vi "Expt5_MT FSK Transceiver_Student_lab.vi"(0 "# Message Symbols":i32=1000, 5 "Eb/N0, dB":dbl(slide)=80.0 scale=0.0..100.0, 9 "Symbol Phase Continuity":enum16{"continuous", "discontinuous"}(ring), 11 "Reset ? (T)":bool=TRUE, 14 "?":T3(tab)=enum."Eye diagram (RX)") -> (3 "FSK System Parameters":T2={"samples per symbol (16)"=4, "symbol map"=[-25000.0, 25000.0], "symbol phase continuity"=enum."continuous"} {"symbol map" format="%.2f"}, 4 "Output Complex Waveform":cluster{"t0":dbl, "dt":dbl, "Y":cdb[]} {"Y" format="%.3f"; "dt" format="%^.2e"; "t0" format="%.4f"}, 6 "Transmitted  Bits":i8[](array[numeric]), 8 "Received Bits":i8[](array[numeric]), 10 "Bit Error Rate":dbl format="%.4e", 13 "Last Sync Found Index":dbl format="%.4f", 15 "Error Out":errorcluster)   [LabVIEW 2020]
doc: "This example demonstrates generation and analysis of FSK modulated signals. You can specify transmit filter parameters, Eb/No, and frequency offset. This example demonstrates programming techniques for resetting the transmitter in cases where the receiver (demodulator) lock is lost. You can also view results of the demodulation on an eye diagram and perform measurements such as bit error rate."
uses:
  <vilib>/addons/Modulation/niDMT.lvlib
  <vilib>/addons/Modulation/niAMT.lvlib
  <vilib>/addons/Modulation/Digital/Support/Controls/FSK System Parameters.ctl
panel:
  out "Estimated Eb/N0(dB)":dbl
  in  "BT":dbl=0.5 format="%.2f"
  out "Current Sampling Rate":dbl=400000.0 format="%.2p"
  in  "Symbol Rate":dbl=100000.0 format="%.2p"
  out "Frequency Offset (Hz)":dbl=-5.3151869530752014e-05 format="%.2f"
  in  "Frequency Offset (Hz)":dbl(slide) scale=-1000.0..1000.0
  in  "FSK Deviation (Hz)":dbl=25000.0 format="%.2p"
  in  "M-FSK":enum16{"2", "4", "8", "16", "32", "64"}(ring)
  in  "TX Filter":T1(ring)=enum."Gaussian"
  out "BER Trigger Found":bool
  in  "Stop":bool
  out "TX Symbols":T4(graph)={{"1/x"=0.0, 1e-05, [1, 1, 0, 1, 0, 1, 1, 0, 1, 0, 0, 1, 1, 1, 1, 1, 1, 1, 0, 1, 0, 0, 0, 1, 0, 1, 1, 0, 0, 0, 1, 1, 1, 0, 1, 0, 1, 1, 0, 0, 1, 0, 1, 1, 0, 0, 1, 1, 1, 1, 0, 0, 0, 1, 1, 1, 1, 1, 0, 1, 1, 1, 0, 1, 0, 0, 0, 0, 0, 1, 1, 0, 1, 0, 1, 1, 0, 1, 1, 0, 1, 1, 1, 0, 1, 1, 0, 0, 0, 0, 0, 1, 0, 1, 1, 0, 1, 0, 1, 1, 1, 1, 1, 0, 1, 0, 1, 0, 1, 0, 1, 0, 0, 0, 0, 0, 0, 1, 0, 1, 0, 0, 1, 0, 1, 0, 1, 1, 1, 1, 0, 0, 1, 0, 1, 1, 1, 0, 1, 1, 1, 0, 0, 0, 0, 0, 0, 1, 1, 1, 0, 0, 1, 1, 1, 0, 1, 0, 0, 1, 0, 0, 1, 1, 1, 1, 0, 1, 0, 1, 1, 1, 0, 1, 0, 1, 0, 0, 0, 1, 0, 0, 1, 0, 0, 0, 0, 1, 1, 0, 0, 1, 1, 1, 0, 0, 0, 0, 1, 0, 1, 1, 1, 1, 0, 1, 1, 0, 1, 1, 0, 0, 1, 1, 0, 1, 0, 0, 0, 0, 1, 1, 1, 0, 1, 1, 1, 1, 0, 0, 0, 0, 1, 1, 1, 1, 1, 1, 1, 1, 1, 0, 0, 0, 0, 0, 1, 1, 1, 1, 0, 1, 1, 1, 1, 1, 0, 0, 0, 1, 0, 1, 1, 1, 0, 0, 1, 1, 0, 0, 1, 0, 0, 0, 0, 0, 1, 0, 0, 1, 0, 1, 0, 0, 1, 1, 1, 0, 1, 1, 0, 1, 0, 0, 0, 1, 1, 1, 1, 0, 0, 1, 1, 1, 1, 1, 0, 0, 1, 1, 0, 1, 1, 0, 0, 0, 1, 0, 1, 0, 1, 0, 0, 1, 0, 0, 0, 1, 1, 1, 0, 0, 0, 1, 1, 0, 1, 1, 0, 1, 0, 1, 0, 1, 1, 1, 0, 0, 0, 1, 0, 0, 1, 1, 0, 0, 0, 1, 0, 0, 0, 1, 0, 0, 0, 0, 0, 0, 0, 0, 1, 0, 0, 0, 0, 1, 0, 0, 0, 1, 1, 0, 0, 0, 0, 1, 0, 0, 1, 1, 1, 0, 0, 1, 0, 1, 0, 1, 0, 1, 1, 0, 0, 0, 0, 1, 1, 0, 1, 1, 1, 1, 0, 1, 0, 0, 1, 1, 0, 1, 1, 1, 0, 0, 1, 0, 0, 0, 1, 0, 1, 0, 0, 0, 0, 1, 0, 1, 0, 1, 1, 0, 1, 0, 0, 1, 1, 1, 1, 1, 1, 0, 1, 1, 0, 0, 1, 0, 0, 1, 0, 0, 1, 0, 1, 1, 0, 1, 1, 1, 1, 1, 1, 0, 0, 1, 0, 0, 1, 1, 0, 1, 0, 1, 0, 0, 1, 1, 0, 0, 1, 1, 0, 0, 0, 0, 0, 0, 0, 1, 1, 0, 0, 0, 1, 1, 0, 0, 1, 0, 1, 0, 0, 0, 1, 1, 0, 1, 0, 0, 1, 0, 1, 1, 1, 1, 1, 1, 1, 0, 1, 0, 0, 0, 1, 0, 1, 1, 0, 0, 0, 1, 1, 1, 0, 1, 0, 1, 1, 0, 0, 1, 0, 1, 1, 0, 0, 1, 1, 1, 1, 0, 0, 0, 1, 1, 1, 1, 1, 0, 1, 1, 1, 0, 1, 0, 0, 0, 0, 0, 1, 1, 0, 1, 0, 1, 1, 0, 1, 1, 0, 1, 1, 1, 0, 1, 1, 0, 0, 0, 0, 0, 1, 0, 1, 1, 0, 1, 0, 1, 1, 1, 1, 1, 0, 1, 0, 1, 0, 1, 0, 1, 0, 0, 0, 0, 0, 0, 1, 0, 1, 0, 0, 1, 0, 1, 0, 1, 1, 1, 1, 0, 0, 1, 0, 1, 1, 1, 0, 1, 1, 1, 0, 0, 0, 0, 0, 0, 1, 1, 1, 0, 0, 1, 1, 1, 0, 1, 0, 0, 1, 0, 0, 1, 1, 1, 1, 0, 1, 0, 1, 1, 1, 0, 1, 0, 1, 0, 0, 0, 1, 0, 0, 1, 0, 0, 0, 0, 1, 1, 0, 0, 1, 1, 1, 0, 0, 0, 0, 1, 0, 1, 1, 1, 1, 0, 1, 1, 0, 1, 1, 0, 0, 1, 1, 0, 1, 0, 0, 0, 0, 1, 1, 1, 0, 1, 1, 1, 1, 0, 0, 0, 0, 1, 1, 1, 1, 1, 1, 1, 1, 1, 0, 0, 0, 0, 0, 1, 1, 1, 1, 0, 1, 1, 1, 1, 1, 0, 0, 0, 1, 0, 1, 1, 1, 0, 0, 1, 1, 0, 0, 1, 0, 0, 0, 0, 0, 1, 0, 0, 1, 0, 1, 0, 0, 1, 1, 1, 0, 1, 1, 0, 1, 0, 0, 0, 1, 1, 1, 1, 0, 0, 1, 1, 1, 1, 1, 0, 0, 1, 1, 0, 1, 1, 0, 0, 0, 1, 0, 1, 0, 1, 0, 0, 1, 0, 0, 0, 1, 1, 1, 0, 0, 0, 1, 1, 0, 1, 1, 0, 1, 0, 1, 0, 1, 1, 1, 0, 0, 0, 1, 0, 0, 1, 1, 0, 0, 0, 1, 0, 0, 0, 1, 0, 0, 0, 0, 0, 0, 0, 0, 1, 0, 0, 0, 0, 1, 0, 0, 0, 1, 1, 0, 0, 0, 0, 1, 0, 0, 1, 1, 1, 0, 0, 1, 0, 1, 0, 1, 0, 1, 1, 0, 0, 0, 0, 1, 1, 0, 1, 1, 1, 1, 0, 1, 0, 0, 1, 1, 0, 1, 1, 1, 0, 0, 1, 0, 0, 0, 1, 0, 1, 0, 0, 0, 0, 1, 0, 1, 0, 1, 1, 0, 1, 0, 0, 1, 1, 1, 1, 1, 1, 0, 1, 1, 0, 0, 1, 0, 0, 1, 0, 0, 1, 0, 1, 1, 0, 1, 1, 1, 1, 1, 1, 0, 0, 1, 0, 0, 1, 1, 0, 1, 0, 1, 0, 0, 1, 1, 0, 0, 1, 1, 0, 0], 1}, [[0]]}
  out "FFT Magnitude (TX)":cluster{dbl, dbl, dbl[]}(graph)={-199609.37499999997, 390.62499999999994, []}
  out "RX Symbols":T4(graph)={{"1/x"=0.0, 1e-05, [1, 1, 0, 1, 0, 1, 1, 0, 1, 0, 0, 1, 1, 1, 1, 1, 1, 1, 0, 1, 0, 0, 0, 1, 0, 1, 1, 0, 0, 0, 1, 1, 1, 0, 1, 0, 1, 1, 0, 0, 1, 0, 1, 1, 0, 0, 1, 1, 1, 1, 0, 0, 0, 1, 1, 1, 1, 1, 0, 1, 1, 1, 0, 1, 0, 0, 0, 0, 0, 1, 1, 0, 1, 0, 1, 1, 0, 1, 1, 0, 1, 1, 1, 0, 1, 1, 0, 0, 0, 0, 0, 1, 0, 1, 1, 0, 1, 0, 1, 1, 1, 1, 1, 0, 1, 0, 1, 0, 1, 0, 1, 0, 0, 0, 0, 0, 0, 1, 0, 1, 0, 0, 1, 0, 1, 0, 1, 1, 1, 1, 0, 0, 1, 0, 1, 1, 1, 0, 1, 1, 1, 0, 0, 0, 0, 0, 0, 1, 1, 1, 0, 0, 1, 1, 1, 0, 1, 0, 0, 1, 0, 0, 1, 1, 1, 1, 0, 1, 0, 1, 1, 1, 0, 1, 0, 1, 0, 0, 0, 1, 0, 0, 1, 0, 0, 0, 0, 1, 1, 0, 0, 1, 1, 1, 0, 0, 0, 0, 1, 0, 1, 1, 1, 1, 0, 1, 1, 0, 1, 1, 0, 0, 1, 1, 0, 1, 0, 0, 0, 0, 1, 1, 1, 0, 1, 1, 1, 1, 0, 0, 0, 0, 1, 1, 1, 1, 1, 1, 1, 1, 1, 0, 0, 0, 0, 0, 1, 1, 1, 1, 0, 1, 1, 1, 1, 1, 0, 0, 0, 1, 0, 1, 1, 1, 0, 0, 1, 1, 0, 0, 1, 0, 0, 0, 0, 0, 1, 0, 0, 1, 0, 1, 0, 0, 1, 1, 1, 0, 1, 1, 0, 1, 0, 0, 0, 1, 1, 1, 1, 0, 0, 1, 1, 1, 1, 1, 0, 0, 1, 1, 0, 1, 1, 0, 0, 0, 1, 0, 1, 0, 1, 0, 0, 1, 0, 0, 0, 1, 1, 1, 0, 0, 0, 1, 1, 0, 1, 1, 0, 1, 0, 1, 0, 1, 1, 1, 0, 0, 0, 1, 0, 0, 1, 1, 0, 0, 0, 1, 0, 0, 0, 1, 0, 0, 0, 0, 0, 0, 0, 0, 1, 0, 0, 0, 0, 1, 0, 0, 0, 1, 1, 0, 0, 0, 0, 1, 0, 0, 1, 1, 1, 0, 0, 1, 0, 1, 0, 1, 0, 1, 1, 0, 0, 0, 0, 1, 1, 0, 1, 1, 1, 1, 0, 1, 0, 0, 1, 1, 0, 1, 1, 1, 0, 0, 1, 0, 0, 0, 1, 0, 1, 0, 0, 0, 0, 1, 0, 1, 0, 1, 1, 0, 1, 0, 0, 1, 1, 1, 1, 1, 1, 0, 1, 1, 0, 0, 1, 0, 0, 1, 0, 0, 1, 0, 1, 1, 0, 1, 1, 1, 1, 1, 1, 0, 0, 1, 0, 0, 1, 1, 0, 1, 0, 1, 0, 0, 1, 1, 0, 0, 1, 1, 0, 0, 0, 0, 0, 0, 0, 1, 1, 0, 0, 0, 1, 1, 0, 0, 1, 0, 1, 0, 0, 0, 1, 1, 0, 1, 0, 0, 1, 0, 1, 1, 1, 1, 1, 1, 1, 0, 1, 0, 0, 0, 1, 0, 1, 1, 0, 0, 0, 1, 1, 1, 0, 1, 0, 1, 1, 0, 0, 1, 0, 1, 1, 0, 0, 1, 1, 1, 1, 0, 0, 0, 1, 1, 1, 1, 1, 0, 1, 1, 1, 0, 1, 0, 0, 0, 0, 0, 1, 1, 0, 1, 0, 1, 1, 0, 1, 1, 0, 1, 1, 1, 0, 1, 1, 0, 0, 0, 0, 0, 1, 0, 1, 1, 0, 1, 0, 1, 1, 1, 1, 1, 0, 1, 0, 1, 0, 1, 0, 1, 0, 0, 0, 0, 0, 0, 1, 0, 1, 0, 0, 1, 0, 1, 0, 1, 1, 1, 1, 0, 0, 1, 0, 1, 1, 1, 0, 1, 1, 1, 0, 0, 0, 0, 0, 0, 1, 1, 1, 0, 0, 1, 1, 1, 0, 1, 0, 0, 1, 0, 0, 1, 1, 1, 1, 0, 1, 0, 1, 1, 1, 0, 1, 0, 1, 0, 0, 0, 1, 0, 0, 1, 0, 0, 0, 0, 1, 1, 0, 0, 1, 1, 1, 0, 0, 0, 0, 1, 0, 1, 1, 1, 1, 0, 1, 1, 0, 1, 1, 0, 0, 1, 1, 0, 1, 0, 0, 0, 0, 1, 1, 1, 0, 1, 1, 1, 1, 0, 0, 0, 0, 1, 1, 1, 1, 1, 1, 1, 1, 1, 0, 0, 0, 0, 0, 1, 1, 1, 1, 0, 1, 1, 1, 1, 1, 0, 0, 0, 1, 0, 1, 1, 1, 0, 0, 1, 1, 0, 0, 1, 0, 0, 0, 0, 0, 1, 0, 0, 1, 0, 1, 0, 0, 1, 1, 1, 0, 1, 1, 0, 1, 0, 0, 0, 1, 1, 1, 1, 0, 0, 1, 1, 1, 1, 1, 0, 0, 1, 1, 0, 1, 1, 0, 0, 0, 1, 0, 1, 0, 1, 0, 0, 1, 0, 0, 0, 1, 1, 1, 0, 0, 0, 1, 1, 0, 1, 1, 0, 1, 0, 1, 0, 1, 1, 1, 0, 0, 0, 1, 0, 0, 1, 1, 0, 0, 0, 1, 0, 0, 0, 1, 0, 0, 0, 0, 0, 0, 0, 0, 1, 0, 0, 0, 0, 1, 0, 0, 0, 1, 1, 0, 0, 0, 0, 1, 0, 0, 1, 1, 1, 0, 0, 1, 0, 1, 0, 1, 0, 1, 1, 0, 0, 0, 0, 1, 1, 0, 1, 1, 1, 1, 0, 1, 0, 0, 1, 1, 0, 1, 1, 1, 0, 0, 1, 0, 0, 0, 1, 0, 1, 0, 0, 0, 0, 1, 0, 1, 0, 1, 1, 0, 1, 0, 0, 1, 1, 1, 1, 1, 1, 0, 1, 1, 0, 0, 1, 0, 0, 1, 0, 0, 1, 0, 1, 1, 0, 1, 1, 1, 1, 1, 1, 0, 0, 1, 0, 0, 1, 1, 0, 1, 0, 1, 0, 0, 1, 1, 0, 0, 1, 1, 0, 0], 1}, [[0]]}
  out "FFT Magnitude (RX)":cluster{dbl, dbl, dbl[]}(graph)={-199899.99999999997, 99.99999999999999, []}
  out "Eye Diagram":cluster{"t0":dbl, "dt":dbl, "Y":dbl[]}[](graph)
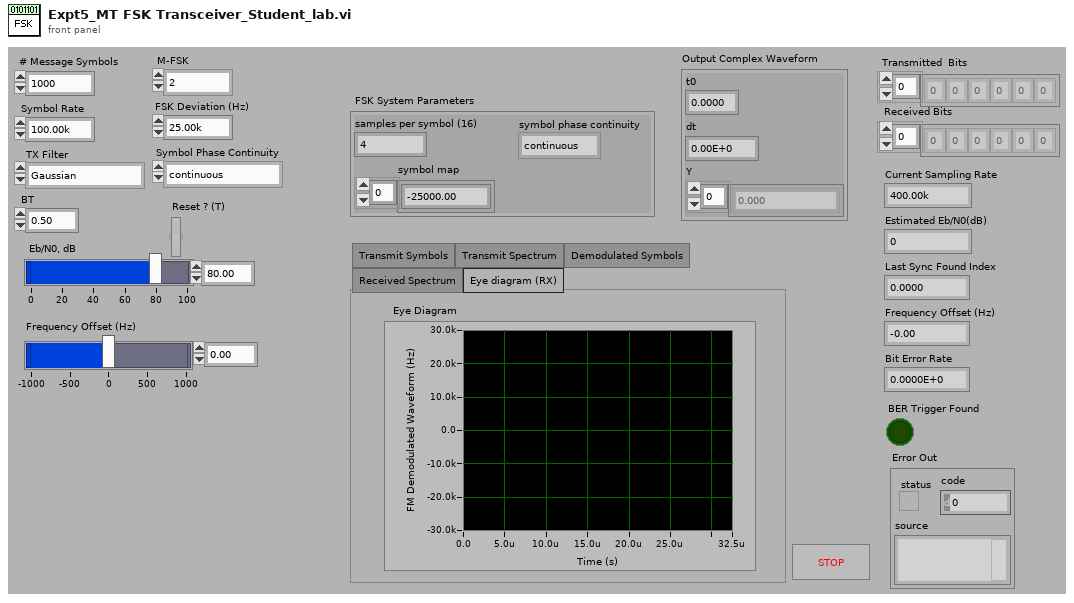
[diagram p1: front panel]
types:
  T1 = enum16{"none", "Raised Cosine", "Root Raised Cos", "Gaussian"}
  T2 = typedef "niDMT.lvlib/FSK System Parameters.ctl" = cluster{"samples per symbol (16)":i32, "symbol map":dbl[], "symbol phase continuity":enum16{"continuous", "discontinuous"}}
  T3 = enum32{"Transmit Symbols", "Transmit Spectrum", "Demodulated Symbols", "Received Spectrum", "Eye diagram (RX)"}
  T4 = cluster{cluster{"1/x":dbl, dbl, i8[], i32}, i32[][]}
  T5 = cluster{"expected sync location (symbols)":i32, "sync sequence":cdb[], "sync location uncertainty (symbols)":i32, "sync indent (symbols)":i32}
  T6 = cluster{"TX Filter":enum16{"none", "Raised Cosine", "Root Raised Cos", "Gaussian"}, "Alpha / BT":dbl, "filter length":i32}
  T7 = cluster{"# Guard Bits":i32, "# Sync Bits":i32, "# Message Bits":i32, "PN sequence order":i32}
  T8 = cluster{"M-FSK":i32, "FSK deviation (Hz)":dbl, "Symbol Phase Continuity":enum16{"continuous", "discontinuous"}}
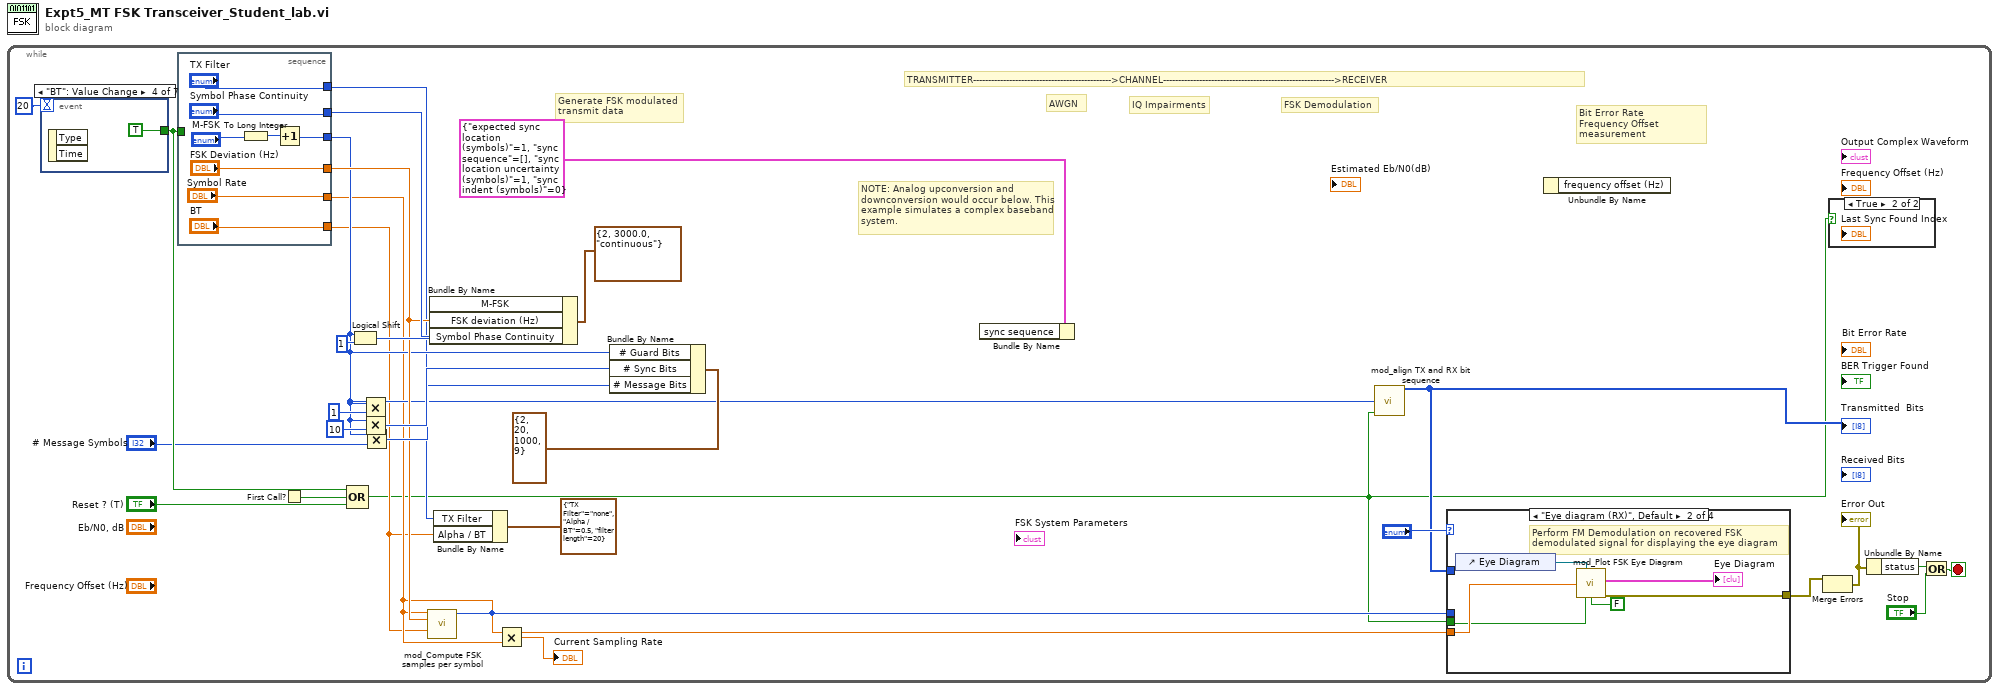
[diagram p0: block diagram]
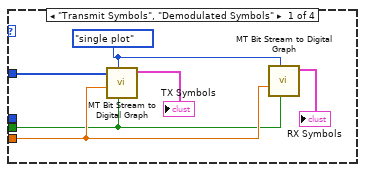
[diagram p3: hidden frame]
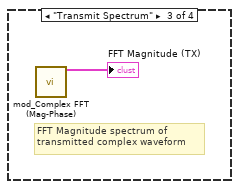
[diagram p4: hidden frame]
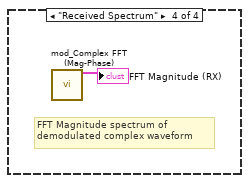
[diagram p5: hidden frame]
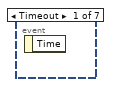
[diagram p6: hidden frame]
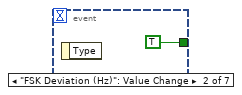
[diagram p7: hidden frame]
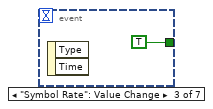
[diagram p8: hidden frame]
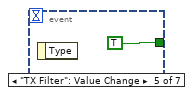
[diagram p9: hidden frame]
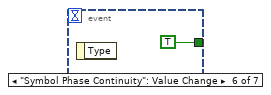
[diagram p10: hidden frame]
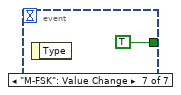
[diagram p11: hidden frame]
diagram:
  n1 = while {
    stop <- w29 stop-if-true
    # "IQ Impairments"
    # "NOTE: Analog upconversion and downconversion would occur below. This example simulates a complex baseband system."
    # "Bit Error Rate\nFrequency Offset\nmeasurement"
    # "AWGN"
    # "TRANSMITTER---------------------------------------------->CHANNEL--------------------------------------------------------->RECEIVER"
    # "Generate FSK modulated\ntransmit data"
    # "FSK Demodulation"
    n2 = event shown="[3] \"BT\": Value Change" {
      selector: _ -> [_ _ _ _ _ _ _]
      dyn-events: _ -> [_ _ _ _ _ _ _]
      timeout: 20 -> [_ _ _ _ _ _ _]
      tunnel: [_ TRUE TRUE TRUE TRUE TRUE TRUE] -> w25
      event Timeout {
        n3 = event-data() -> ()  [unwired: 1 in, 1 out]
      }
      event "FSK Deviation (Hz)": Value Change {
        n4 = event-data() -> ()  [unwired: 1 in, 1 out]
      }
      event "Symbol Rate": Value Change {
        n5 = event-data() -> ()  [unwired: 1 in, 2 out]
      }
      event "BT": Value Change {
        n6 = event-data() -> ()  [unwired: 1 in, 2 out]
      }
      event "TX Filter": Value Change {
        n7 = event-data() -> ()  [unwired: 1 in, 1 out]
      }
      event "Symbol Phase Continuity": Value Change {
        n8 = event-data() -> ()  [unwired: 1 in, 1 out]
      }
      event "M-FSK": Value Change {
        n9 = event-data() -> ()  [unwired: 1 in, 1 out]
      }
    }
    n10 = stacked-sequence {
      tunnel: w25 -> [_]
      tunnel: ["TX Filter"] -> w5
      tunnel: ["Symbol Phase Continuity"] -> w20
      tunnel: [w50] -> w9
      tunnel: ["FSK Deviation (Hz)"] -> w10
      tunnel: ["Symbol Rate"] -> w8
      tunnel: ["BT"] -> w4
      frame #0 {
        n11 = To Long Integer(number="M-FSK") -> (32bit integer=w49:i32)
        n12 = Increment(x=w49) -> (x+1=w50:i32)
      }
    }
    n13 = First Call?() -> (First Call?: T/F=w26:bool)
    n14 = Compound Arithmetic op=OR(w25, w26, "Reset ? (T)") -> (w1:bool)
    n15 = Logical Shift(y=w9, x=1) -> (x << y=w21:i32)
    n16 = Multiply(x=w9, y=1) -> ()  [unwired: 1 out]
    n17 = Multiply(x=w9, y=10) -> (x*y=w15:i32)
    n18 = Multiply(x=w9, y="# Message Symbols") -> (x*y=w14:i32)
    n19 = call <vilib>:"mod_Compute FSK samples per symbol.vi"("Symbol Rate"=w8, "Deviation (Hz)"=w10, "Filter parameter"=w4) -> ("FSK samples per symbol"=w3:i32)  [unwired: 11 in, 1 out]
    n20 = Bundle By Name(cluster=T8 {"M-FSK"=2, "FSK deviation (Hz)"=3000.0, "Symbol Phase Continuity"=enum."continuous"} ("FSK Specific"), "M-FSK"=w21, "FSK deviation (Hz)"=w10, "Symbol Phase Continuity"=w20) -> ()  [unwired: 1 out]
    n21 = Bundle By Name(cluster=T6 {"TX Filter"=enum."none", "Alpha / BT"=0.5, "filter length"=20} ("System Filter"), "TX Filter"=w5, "Alpha / BT"=w4) -> ()  [unwired: 1 out]
    n22 = Multiply(x=w3, y=w8) -> (x*y=→"Current Sampling Rate":dbl)
    n23 = Bundle By Name(cluster=T7 {"# Guard Bits"=2, "# Sync Bits"=20, "# Message Bits"=1000, "PN sequence order"=9} ("Message"), "# Guard Bits"=w9, "# Sync Bits"=w15, "# Message Bits"=w14) -> ()  [unwired: 1 out]
    n24 = Bundle By Name(cluster=T5 {"expected sync location (symbols)"=1, "sync sequence"=[], "sync location uncertainty (symbols)"=1, "sync indent (symbols)"=0} ("synchronization parameters")) -> ()  [unwired: 1 in, 1 out]
    n25 = call <vilib>:"mod_align TX and RX bit sequence.vi"("# Bits removed"=w9, "Reset"=w1) -> ("Aligned array"=w13:i8[])  [unwired: 13 in]
    "Transmitted  Bits" <- w13
    n26 = case shown="\"Eye diagram (RX)\", Default" "?" {
      tunnel: w8 -> [w35 w43 _ _]
      tunnel: w3 -> [_ _ _ _]
      tunnel: w13 -> [w34 _ _ _]
      tunnel: [_ w41 _ _] -> w12
      tunnel: w1 -> [w32 w38 _ _]
      frame "Transmit Symbols", "Demodulated Symbols" {
        w36 = enum16{"single plot", "plot per bit"}."single plot" ("Format")
        n27 = call <vilib>:"MT Bit Stream to Digital Graph.vi"("Reset (F)"=w32, "Format"=w36, "Symbol Rate (Hz)"=w35, "Bit Stream"=w34) -> ("Digital Waveform Graph"=→"TX Symbols":T4)  [unwired: 7 in]
        n28 = call <vilib>:"MT Bit Stream to Digital Graph.vi"("Reset (F)"=w32, "Format"=w36, "Symbol Rate (Hz)"=w35) -> ("Digital Waveform Graph"=→"RX Symbols":T4)  [unwired: 8 in]
      }
      frame "Eye diagram (RX)", Default {
        # "Perform FM Demodulation on recovered FSK\ndemodulated signal for displaying the eye diagram"
        n29 = control-ref of="Eye Diagram"() -> (w42:refnum<vi>)
        n30 = call <vilib>:"mod_Plot FSK Eye Diagram.vi"("Rx Eye Diagram"=w42, "autoscale"=FALSE, "Symbol Rate, Hz"=w43, "Reset?"=w38) -> ("FSK Eye Diagram"=→"Eye Diagram":cluster{"t0":dbl, "dt":dbl, "Y":dbl[]}[], "error out"=w41:errorcluster)  [unwired: 9 in, 1 out]
      }
      frame "Transmit Spectrum" {
        # "FFT Magnitude spectrum of \ntransmitted complex waveform"
        n31 = call <vilib>:"mod_Complex FFT (Mag-Phase).vi"() -> ("Magnitude"=→"FFT Magnitude (TX)":cluster{"f0":dbl, "df":dbl, "Y":dbl[]})  [unwired: 14 in, 1 out]
      }
      frame "Received Spectrum" {
        # "FFT Magnitude spectrum of\ndemodulated complex waveform"
        n32 = call <vilib>:"mod_Complex FFT (Mag-Phase).vi"() -> ("Magnitude"=→"FFT Magnitude (RX)":cluster{"f0":dbl, "df":dbl, "Y":dbl[]})  [unwired: 14 in, 1 out]
      }
    }
    n33 = Unbundle By Name() -> ()  [unwired: 1 in, 1 out]
    n34 = Merge Errors(w12) -> (w11:errorcluster)  [unwired: 1 in]
    "Error Out" <- w11
    n35 = case shown="True" w1 {
      frame False {
      }
      frame True {
      }
    }
    n36 = Unbundle By Name(w11) -> ("status"=w31:bool)
    n37 = Or(x=w31, y="Stop") -> (x .or. y?=w29:bool)
  }
